vi "Untitled 6 (SubVI).vi"(9 "increment":bool, 10 "Numeric":i32, 11 "MagAnalysis_Online in":refnum<class "MagAnalysis_Online.lvclass">) -> (1 "B [T]":dbl, 2 "Cluster":T1, 3 "MagAnalysis_Online out":refnum<class "MagAnalysis_Online.lvclass">, 4 "time":u32)   [LabVIEW 2011, in "MagAnalysis_Online.lvclass"]
uses:
  MagAnalysis_Online.lvclass
  MagAnalysis_Online.lvclass/MagAnalysis_Online.ctl
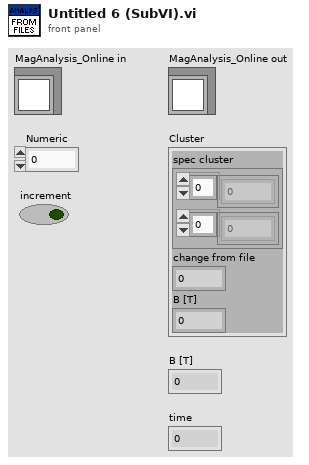
[diagram p1: front panel]
types:
  T1 = cluster{"spec cluster":cluster{dbl[], dbl[]}, "change from file":dbl, "B [T]":dbl}
  T2 = typedef "MagAnalysis_Online.lvclass/analysis_data_typdef.ctl" = cluster{"cam0":T3, "cam1":T3, "cam2":T3, "cam3":T3}
  T3 = typedef "IMAQ Image.ctl" = refnum<image>
  T4 = typedef "bgImages_tyudef.ctl" = cluster{"cam 0":T3, "cam 1":T3, "cam 2":T3, "cam 3":T3}
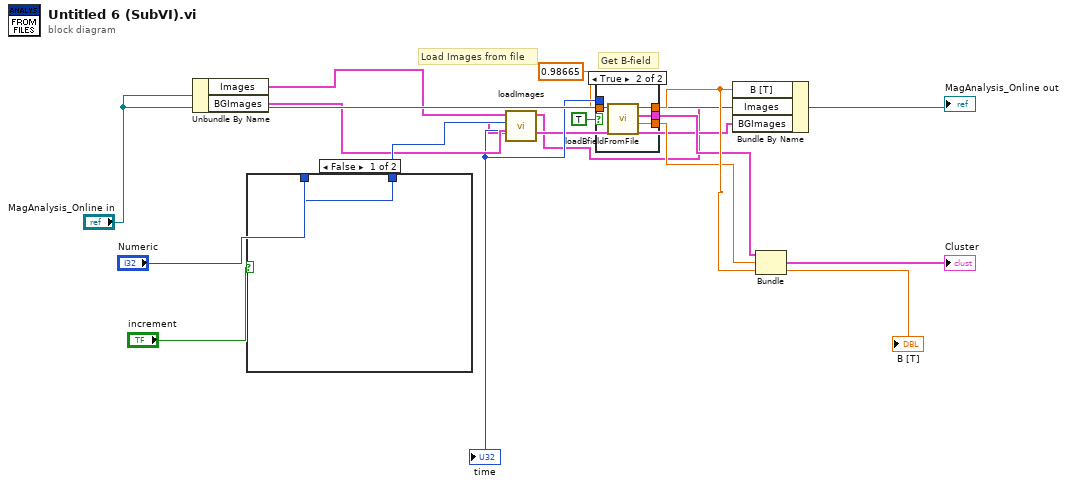
[diagram p0: block diagram]
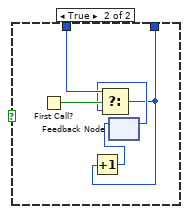
[diagram p2: hidden frame]
diagram:
  # "Get B-field"
  # "Load Images from file"
  n1 = Unbundle By Name("MagAnalysis_Online in") -> ("Images"=w7:T2, "BGImages"=w8:T4)
  n2 = case shown="False" "increment" {
    tunnel: "Numeric" -> [w17 w21]
    tunnel: [w17 w18] -> w10
    frame False {
    }
    frame True {
      n3 = First Call?() -> (First Call?: T/F=w22:bool)
      n4 = feedback #1() -> (w19:i32)  [unwired: 1 in]
      n5 = Select(t=w21, s=w22, f=w19) -> (s? t:f=w18:i32)
      n6 = Increment(x=w18) -> (x+1=w20:i32)
      n7 = feedback-in #1(w20) -> ()
    }
  }
  n8 = call "loadImages.vi"("BGImages"=w8, "Numeric"=w10, "data"=w7) -> ("time"=w5:u32, "BG Images out"=w2:T4, "dat6a out"=w1:T2)  [unwired: 6 in]
  "time" <- w5
  n9 = case shown="True" TRUE {
    tunnel: [w23 w27] -> w15
    tunnel: 0.98665 ("B [T] 2") -> [w23 _]
    tunnel: [_ w26] -> w13
    tunnel: w5 -> [_ w25]
    tunnel: [_ w24] -> w14
    frame False {
    }
    frame True {
      n10 = call "loadBfieldFromFile.vi"("index"=w25) -> ("change from file"=w24:dbl, "spec cluster"=w26:cluster{dbl[], dbl[]}, "B [T]"=w27:dbl)  [unwired: 8 in]
    }
  }
  "B [T]" <- w15
  n11 = Bundle By Name(cluster="MagAnalysis_Online in", "B [T]"=w15, "Images"=w1, "BGImages"=w2) -> (→"MagAnalysis_Online out":refnum<class "MagAnalysis_Online.lvclass">)
  n12 = Bundle("spec cluster"=w13, "change from file"=w14, "B [T]"=w15) -> (→"Cluster":T1)  [unwired: 1 in]
